vi "AlliGator Save Calibration Phasor Map.vi"(8 "Error In":errorcluster, 10 "File Path (empty: dialog)":path=path "", 11 "Calibration Phasor Map":T1={"Phasor Frequency"=80000000.0, "Calibration Lifetime"=1e-09, "ROI Centers"=[], "ROI Descriptors"=[], "Map Resolution X"=0, "Map Resolution Y"=0, "z Array"=[]} {"ROI Descriptors"."Contours"."Type" items=["No Selection", "Point", "Line", "Rectangle", "Oval", "Polygon", "Freehand Region", "Annulus", "Unused2", "Unused3", "Broken Line", "Freehand Line", "Rotated Rectangle"]}) -> (0 "error out":errorcluster, 1 "Message":string, 2 "File Path":path)   [LabVIEW 2021, in "AlliGator Phasor Calibration.lvlib"]
doc: "Saves the <B>Phasor Calibration Map</B>."
uses:
  AlliGator Phasor Calibration.lvlib
  Phasor/Phasor Calibration Map v2.ctl
  e45a3084-940c-4ec1-8177-cb3d35e17e80.vi
  <vilib>/JDP Science/JSONtext/Variant to JSON Text.vi
  <vilib>/JDP Science/JSONtext/LVClass Serializer/JSONtext LVClass Serializer.lvclass
  Phasor/Phasor.lvlib
panel:
  # "see the AlliGator License on the block diagram (Ctrl+E or Window:Show Block Diagram)"
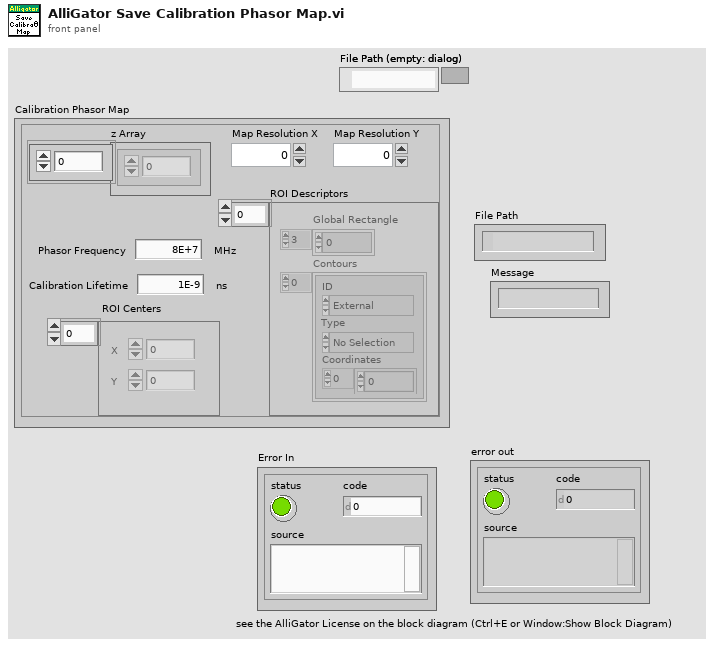
[diagram p1: front panel]
types:
  T1 = typedef "Phasor.lvlib/Phasor Calibration Map v2.ctl" = cluster{"Phasor Frequency":dbl[unit], "Calibration Lifetime":dbl[unit], "ROI Centers":cluster{"X":i32, "Y":i32}[], "ROI Descriptors":T2[], "Map Resolution X":i32, "Map Resolution Y":i32, "z Array":cdb[]}
  T2 = typedef "ROI Descriptor" = cluster{"Global Rectangle":i32[], "Contours":cluster{"ID":enum32{"External", "Internal"}, "Type":u32, "Coordinates":i32[]}[]}
  T3 = typedef "AlliGator Phasor Calibration.lvlib/AlliGator Phasor Calibration Map v1.ctl" = cluster{"m Array":dbl[], "phi Array":dbl[], "Phasor Frequency":dbl[unit], "Calibration Lifetime":dbl[unit], "ROI Centers":cluster{"X":i32, "Y":i32}[], "ROI Descriptors":T2[], "Map Resolution X":i32, "Map Resolution Y":i32}
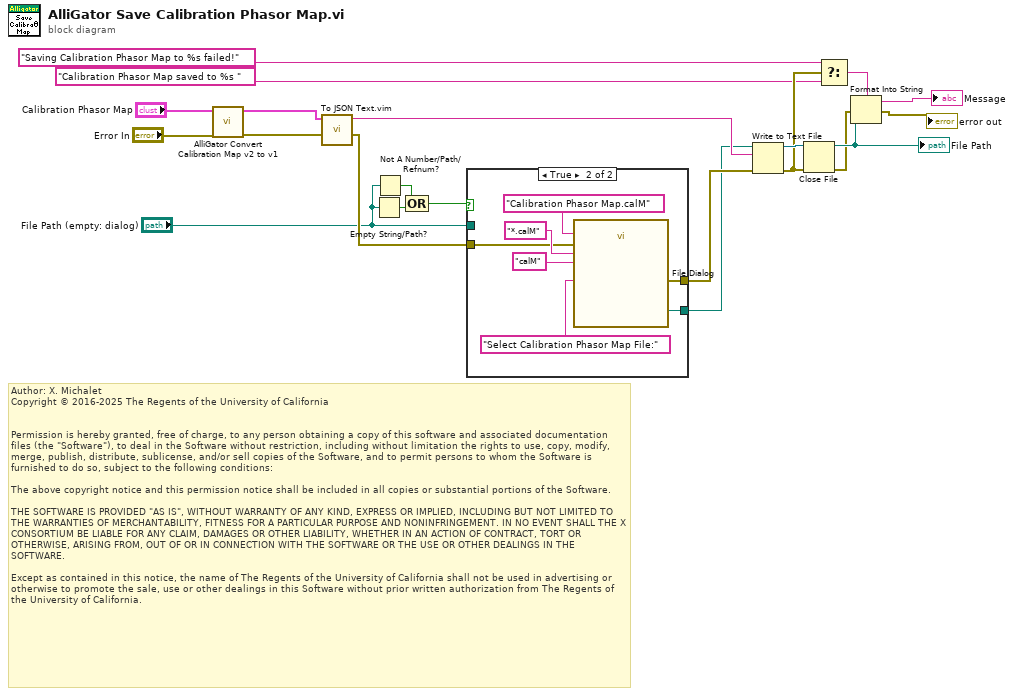
[diagram p0: block diagram]
diagram:
  # "Author: X. Michalet\nCopyright © 2016-2025 The Regents of the University of California\n \n\nPermission is hereby granted, free of charge, to any person obtaining a copy of this software and associated documentation files (the \"Software\"), to deal in the Software without restriction, including without limitation the rights to use, copy, modify, merge, publish, distribute, sublicense, and/or sell copies of the Software, and to permit persons to whom the Software is furnished to do so, subject to the following conditions:\n\nThe above copyright notice and this permission notice shall be included in all copies or substantial portions of the Software.\n\nTHE SOFTWARE IS PROVIDED \"AS IS\", WITHOUT WARRANTY OF ANY KIND, EXPRESS OR IMPLIED, INCLUDING BUT NOT LIMITED TO THE WARRANTIES OF MERCHANTABILITY, FITNESS FOR A PARTICULAR PURPOSE AND NONINFRINGEMENT. IN NO EVENT SHALL THE X CONSORTIUM BE LIABLE FOR ANY CLAIM, DAMAGES OR OTHER LIABILITY, WHETHER IN AN ACTION OF CONTRACT, TORT OR OTHERWISE, ARISING FROM, OUT OF OR IN CONNECTION WITH THE SOFTWARE OR THE USE OR OTHER DEALINGS IN THE SOFTWARE.\n\nExcept as contained in this notice, the name of The Regents of the University of California shall not be used in advertising or otherwise to promote the sale, use or other dealings in this Software without prior written authorization from The Regents of the University of California."
  n1 = call "AlliGator Convert Calibration Map v2 to v1.vi"("error in (no error)"="Error In", "Calibration Phasor Map v2"="Calibration Phasor Map") -> ("error out"=w4:errorcluster, "Phasor Calibration Map v1"=w5:T3)  [unwired: 8 in]
  n2 = call "To JSON Text.vim"("error in (no error)"=w4, "Anything"=w5) -> ("error out"=w18:errorcluster, "<JSON>"=w15:string)  [unwired: 8 in]
  n3 = Empty String/Path?(string/path="File Path (empty: dialog)") -> (empty?=w9:bool)
  n4 = Not A Number/Path/Refnum?(number/path/refnum="File Path (empty: dialog)") -> (NaN/Path/Refnum?=w1:bool)
  n5 = Compound Arithmetic op=OR(w1, w9) -> (w2:bool)
  n6 = case shown="True" w2 {
    tunnel: w18 -> [w23 w27]
    tunnel: [w23 w25] -> w16
    tunnel: [w22 w24] -> w14
    tunnel: "File Path (empty: dialog)" -> [w22 _]
    frame False {
    }
    frame True {
      n7 = call "File Dialog"("prompt"="Select Calibration Phasor Map File:" ("Prompt"), "default name"="Calibration Phasor Map.calM", "error in"=w27, "pattern (all files)"="*.calM" ("Pattern (*.xml;*.XML)"), "pattern label"="calM" ("File Extension (xml)")) -> ("selected path"=w24:path, "error out"=w25:errorcluster)  [unwired: 7 in, 2 out]
    }
  }
  n8 = Write to Text File(file (use dialog)=w14, text=w15, error in=w16) -> (refnum out=w17:refnum<file>, error out=w12:errorcluster)  [unwired: 1 in, 1 out]
  n9 = Close File(refnum=w17, error in=w12) -> (path=w13:path, error out=w8:errorcluster)
  "File Path" <- w13
  n10 = Select(t="Saving Calibration Phasor Map to %s failed!" ("format string"), s=w12, f="Calibration Phasor Map saved to %s " ("format string")) -> (s? t:f=w21:string)
  n11 = Format Into String(format string=w21, error in=w8, w13) -> (resulting string=→"Message":string, error out=→"error out":errorcluster)  [unwired: 1 in]
